vi "RT-FPGA9213.vi"(8 "错误输入":errorcluster, 9 "9213dt输入":dbl, 11 "FPGA VI引用输入":refnum<k20>) -> (0 "错误输出":errorcluster, 1 "9213dt 输出":dbl, 2 "9213输出数组":dbl[](array[numeric]), 3 "FPGA VI引用输出":refnum<k20>, 4 "9213t0":timestamp, 5 "9213数据波形":waveform(dbl) caption="输出波形")   [LabVIEW 2013]
uses:
  D:/labview/ni.anzhuang/LabVIEW 2013/examples/CompactRIO/Shared/cRIO Convert Thermocouple Readings.llb/Thermocouple Type.ctl
  <vilib>/rvi/interface/common/niFpgaWaitOnOcc.vi
  <vilib>/Utility/error.llb/Error Cluster From Error Code.vi
  <vilib>/rvi/errors/niLvFpgaAdjustHostInterfaceError.vi
  D:/labview/ni.anzhuang/LabVIEW 2013/examples/CompactRIO/Module Specific/NI 9213/NI 9213 Support Files.llb/NI 9213 Convert to Temperature (Calibrated).vi
  <vilib>/rvi/interface/nirviMethod/nirviMethod.xnode
  <vilib>/rvi/interface/nirviReadWriteControl/nirviReadWriteControl.xnode
  NiFpgaLv.dll
  <vilib>/rvi/interface/Simulation/niFpgaSimulationCallBeginRW.vi
  <vilib>/rvi/interface/nirviMethod/StockFPGA_InlinedMethodWaitForSingleIRQ.vi
  <vilib>/FPGAPlugInAG/Dynamic/niLvFpga_WaitOnIrq_Dynamic.vi
  <vilib>/FPGAPlugInAG/Dynamic/niLvFpga_AcknowledgeIrq_Dynamic.vi
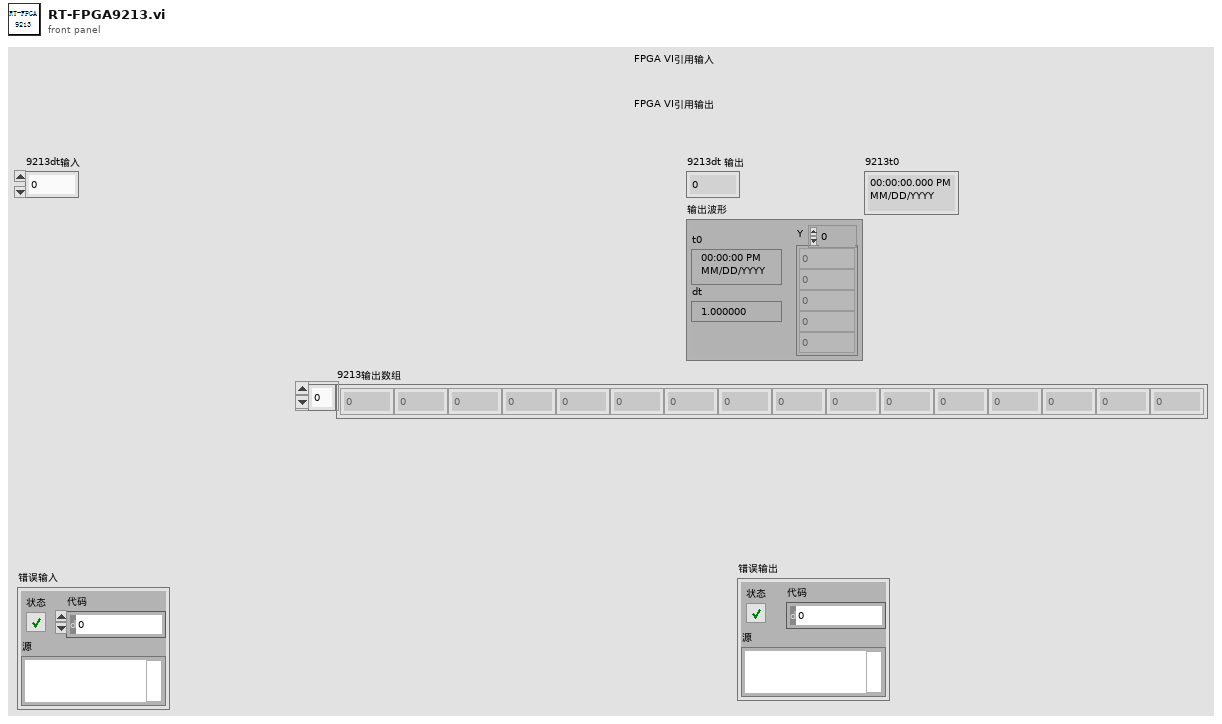
[diagram p1: front panel]
types:
  T1 = typedef "Thermocouple Type.ctl" = u16
  T2 = cluster{"模块6/Autozero":fxp<+/-,24,-2>, "模块6/CJC":fxp<+/-,24,-2>, "模块6/TC0":fxp<+/-,24,-2>, "模块6/TC1":fxp<+/-,24,-2>, "模块6/TC2":fxp<+/-,24,-2>, "模块6/TC3":fxp<+/-,24,-2>, "模块6/TC4":fxp<+/-,24,-2>, "模块6/TC5":fxp<+/-,24,-2>, "模块6/TC6":fxp<+/-,24,-2>, "模块6/TC7":fxp<+/-,24,-2>, "模块6/TC8":fxp<+/-,24,-2>, "模块6/TC9":fxp<+/-,24,-2>, "模块6/TC10":fxp<+/-,24,-2>, "模块6/TC11":fxp<+/-,24,-2>, "模块6/TC12":fxp<+/-,24,-2>, "模块6/TC13":fxp<+/-,24,-2>, "模块6/TC14":fxp<+/-,24,-2>, "模块6/TC15":fxp<+/-,24,-2>}
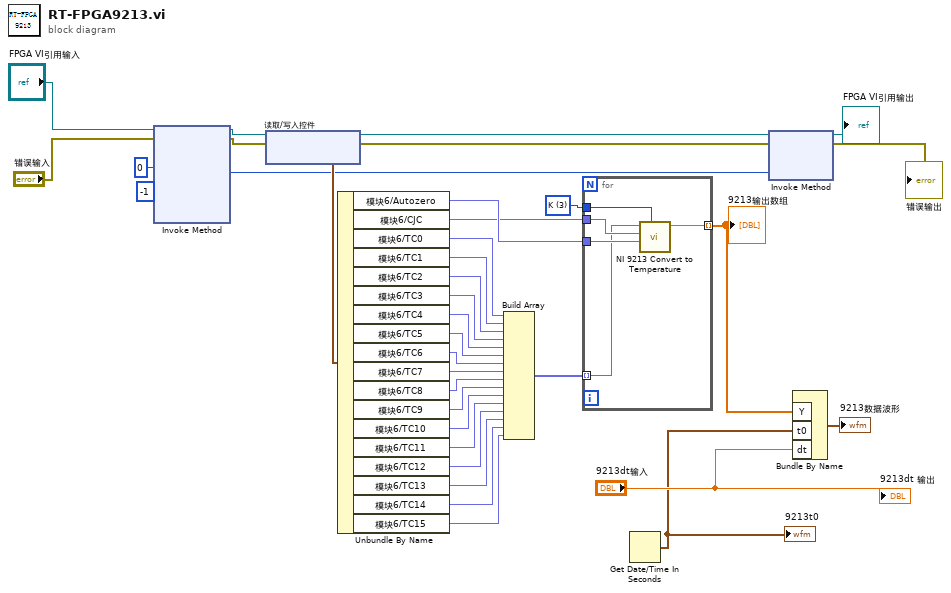
[diagram p0: block diagram]
diagram:
  w36 = T1 3 items=["B", "E", "J", "K", "R", "S", "T", "N"] ("ThermocoupleType")
  n1 = xnode "Invoke Method"("FPGA VI引用输入"="FPGA VI引用输入", "错误输入"="错误输入", "IRQ编号"=0, "超时(ms)"=-1) -> ("FPGA VI引用输出"=w14:refnum<k20>, "错误输出"=w13:errorcluster, "IRQ置有效"=w9:i32)  [unwired: 1 out]
  n2 = xnode "读取/写入控件"("FPGA VI引用输入"=w14, "错误输入"=w13) -> ("FPGA VI引用输出"=w35:refnum<k20>, "错误输出"=w10:errorcluster, "9213输出数据"=w34:T2)
  n3 = Unbundle By Name(w34) -> ("模块6/Autozero"=w33:fxp<+/-,24,-2>, "模块6/CJC"=w32:fxp<+/-,24,-2>, "模块6/TC0"=w31:fxp<+/-,24,-2>, "模块6/TC1"=w30:fxp<+/-,24,-2>, "模块6/TC2"=w29:fxp<+/-,24,-2>, "模块6/TC3"=w28:fxp<+/-,24,-2>, "模块6/TC4"=w27:fxp<+/-,24,-2>, "模块6/TC5"=w26:fxp<+/-,24,-2>, "模块6/TC6"=w25:fxp<+/-,24,-2>, "模块6/TC7"=w24:fxp<+/-,24,-2>, "模块6/TC8"=w23:fxp<+/-,24,-2>, "模块6/TC9"=w22:fxp<+/-,24,-2>, "模块6/TC10"=w21:fxp<+/-,24,-2>, "模块6/TC11"=w20:fxp<+/-,24,-2>, "模块6/TC12"=w19:fxp<+/-,24,-2>, "模块6/TC13"=w18:fxp<+/-,24,-2>, "模块6/TC14"=w17:fxp<+/-,24,-2>, "模块6/TC15"=w16:fxp<+/-,24,-2>)
  n4 = Build Array(w31, w30, w29, w28, w27, w26, w25, w24, w23, w22, w21, w20, w19, w18, w17, w16) -> (w15:fxp<+/-,24,-2>[])
  n5 = for {
    tunnel: w36 -> [w41]
    tunnel: [w40] -> w6 mode=indexing
    tunnel: w33 -> [w39]
    tunnel: w32 -> [w38]
    tunnel: w15 -> [w37] mode=indexing
    n6 = call-poly "NI 9213 Convert to Temperature.vi"("ThermocoupleType"=w41, "AutoZero"=w39, "CJC"=w38, "TC Input"=w37) -> ("Thermocouple Temperature"=w40:dbl)  [unwired: 1 in, 6 out]
  }
  "9213输出数组" <- w6
  n7 = Get Date/Time In Seconds() -> (seconds since 1Jan1904=w4:timestamp)
  "9213t0" <- w4
  n8 = xnode "Invoke Method"("FPGA VI引用输入"=w35, "错误输入"=w10, "IRQ编号"=w9) -> ("FPGA VI引用输出"=→"FPGA VI引用输出":refnum<k20>, "错误输出"=→"错误输出":errorcluster)
  n9 = Bundle By Name("Y"=w6, "t0"=w4, "dt"="9213dt输入") -> (→"9213数据波形":waveform(dbl))  [unwired: 1 in]
  "9213dt 输出" <- "9213dt输入"
